vi "set current(without frequency).vi"(0 "源":i32, 5 "仪器设置":T2, 7 "电流":dbl, 9 "参考信号":T1, 11 "电阻":dbl) -> (10 "电压":dbl)   [LabVIEW 2019, in "old.lvlib"]
uses:
  lib/Keithley 622x/Configure/6221 Wave/Low Level/Typedefs/KE6221 -- Wave Type.ctl
  lib/Keithley 622x/Configure/6221 Wave/Low Level/Typedefs/KE6221 -- Wave Ranging Mode.ctl
  lib/Keithley 622x/Configure/6221 Wave/Low Level/Typedefs/KE6221 -- Wave Playback Time.ctl
  lib/Keithley 622x/Configure/Source/Typedefs/KE622x -- Current Level.ctl
  old.lvlib
  lib/Stanford Research 830/Stanford Research 830.lvlib
  lib/Keithley 622x/Keithley 622x.lvlib
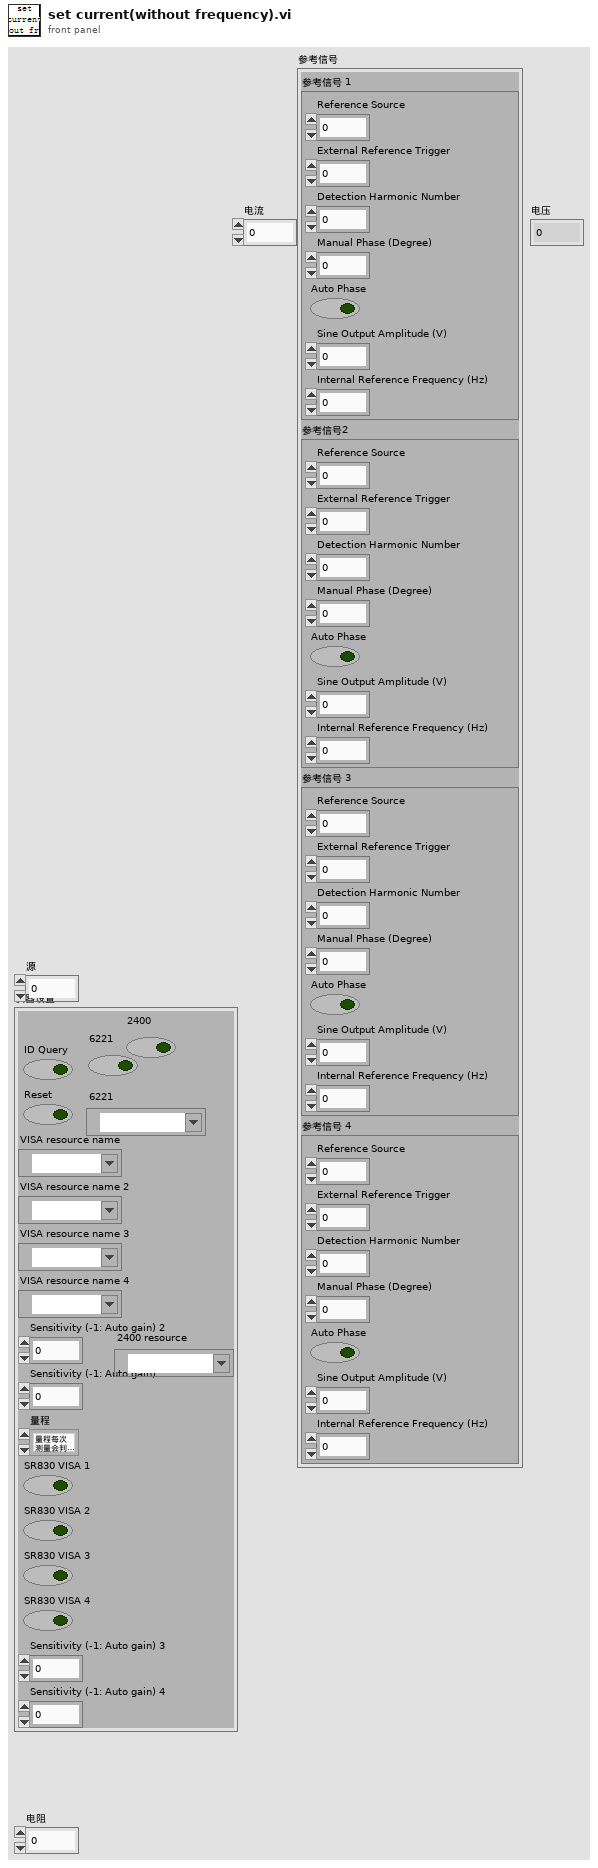
[diagram p1: front panel]
types:
  T1 = cluster{"参考信号 1":cluster{"Reference Source":u16, "External Reference Trigger  ":u16, "Detection Harmonic Number ":dbl, "Manual Phase (Degree)":dbl, "Auto Phase ":bool, "Sine Output Amplitude (V)":dbl, "Internal Reference Frequency (Hz)":dbl}, "参考信号2":cluster{"Reference Source":u16, "External Reference Trigger  ":u16, "Detection Harmonic Number ":dbl, "Manual Phase (Degree)":dbl, "Auto Phase ":bool, "Sine Output Amplitude (V)":dbl, "Internal Reference Frequency (Hz)":dbl}, "参考信号 3":cluster{"Reference Source":u16, "External Reference Trigger  ":u16, "Detection Harmonic Number ":dbl, "Manual Phase (Degree)":dbl, "Auto Phase ":bool, "Sine Output Amplitude (V)":dbl, "Internal Reference Frequency (Hz)":dbl}, "参考信号 4":cluster{"Reference Source":u16, "External Reference Trigger  ":u16, "Detection Harmonic Number ":dbl, "Manual Phase (Degree)":dbl, "Auto Phase ":bool, "Sine Output Amplitude (V)":dbl, "Internal Reference Frequency (Hz)":dbl}}
  T2 = cluster{"ID Query":bool, "Reset":bool, "VISA resource name":refnum<visa-resource-name>, "VISA resource name 2":refnum<visa-resource-name>, "VISA resource name 3":refnum<visa-resource-name>, "VISA resource name 4":refnum<visa-resource-name>, "Sensitivity (-1: Auto gain) 2":i16, "Sensitivity (-1: Auto gain)":i16, "量程":enum16{"量程每次测量会判定", "量程不变为设定值"}, "SR830 VISA 1":bool, "SR830 VISA 2":bool, "SR830 VISA 3":bool, "SR830 VISA 4":bool, "Sensitivity (-1: Auto gain) 3":i16, "Sensitivity (-1: Auto gain) 4":i16, "6221":bool, "6221":refnum<visa-resource-name>, "2400":bool, "2400 resource":refnum<visa-resource-name>}
  T3 = cluster{"Reference Source":u16, "External Reference Trigger  ":u16, "Detection Harmonic Number ":dbl, "Manual Phase (Degree)":dbl, "Auto Phase ":bool, "Sine Output Amplitude (V)":dbl, "Internal Reference Frequency (Hz)":dbl}
  T4 = typedef "Keithley 622x.lvlib/KE622x -- Current Level.ctl" = dbl
  T5 = typedef "Keithley 622x.lvlib/KE6221 -- Wave Playback Time.ctl" = dbl
  T6 = typedef "Keithley 622x.lvlib/KE6221 -- Wave Ranging Mode.ctl" = enum16{"Best", "Fixed"}
  T7 = typedef "Keithley 622x.lvlib/KE6221 -- Wave Type.ctl" = enum16{"Sinusoid", "Square", "Ramp", "Arbitrary 0", "Arbitrary 1", "Arbitrary 2", "Arbitrary 3", "Arbitrary 4"}
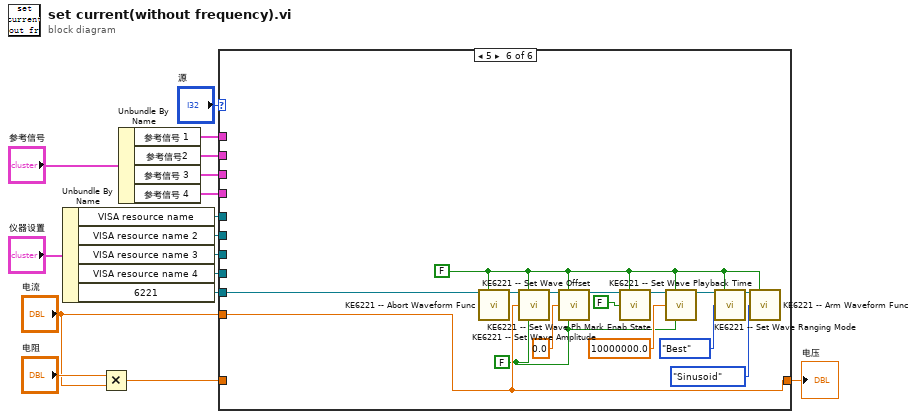
[diagram p0: block diagram]
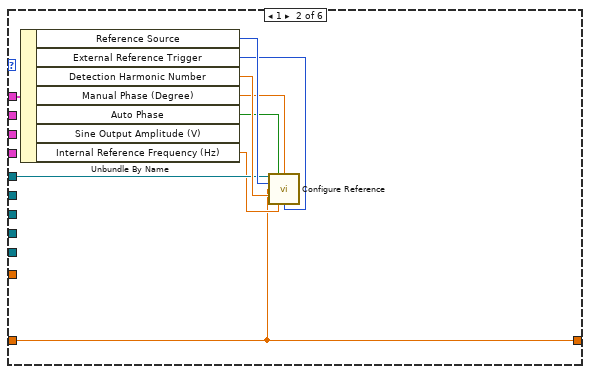
[diagram p3: hidden frame]
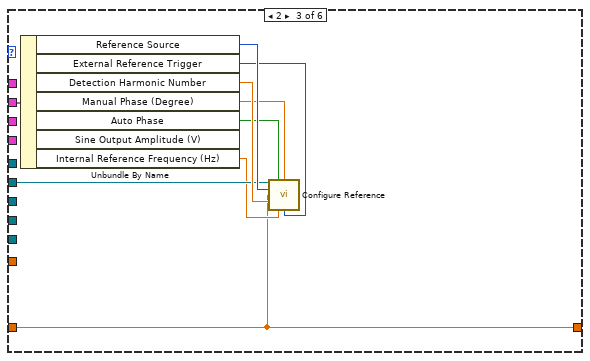
[diagram p4: hidden frame]
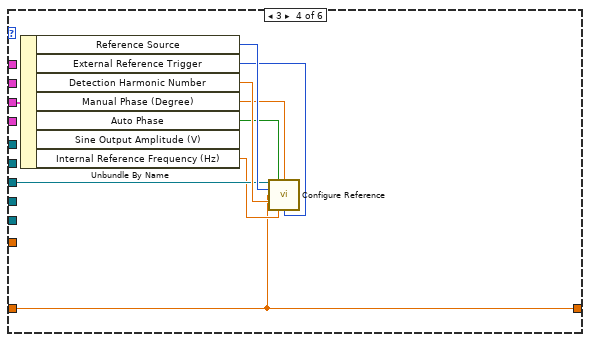
[diagram p5: hidden frame]
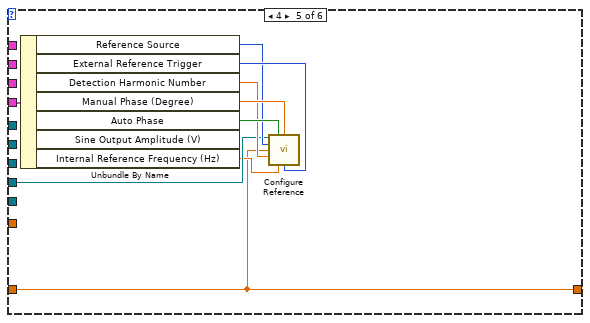
[diagram p6: hidden frame]
diagram:
  n1 = Unbundle By Name("仪器设置") -> ("VISA resource name"=w12:refnum<visa-resource-name>, "VISA resource name 2"=w15:refnum<visa-resource-name>, "VISA resource name 3"=w14:refnum<visa-resource-name>, "VISA resource name 4"=w13:refnum<visa-resource-name>, "6221"=w3:refnum<visa-resource-name>)
  n2 = Multiply(x="电阻", y="电流") -> (x*y=w11:dbl)
  n3 = Unbundle By Name("参考信号") -> ("参考信号 1"=w7:T3, "参考信号2"=w5:T3, "参考信号 3"=w4:T3, "参考信号 4"=w6:T3)
  n4 = case shown="5" "源" {
    tunnel: w11 -> [w17 w18 w27 w36 w45 _]
    tunnel: w12 -> [_ w21 _ _ _ _]
    tunnel: w13 -> [_ _ _ _ w48 _]
    tunnel: w14 -> [_ _ _ w39 _ _]
    tunnel: w15 -> [_ _ w30 _ _ _]
    tunnel: w7 -> [_ w20 _ _ _ _]
    tunnel: w5 -> [_ _ w29 _ _ _]
    tunnel: w4 -> [_ _ _ w38 _ _]
    tunnel: w6 -> [_ _ _ _ w47 _]
    tunnel: w3 -> [_ _ _ _ _ w66]
    tunnel: "电流" -> [_ _ _ _ _ w68]
    tunnel: [w17 w18 w27 w36 w45 w68] -> w1
    frame 0, Default {
    }
    frame 1 {
      n5 = Unbundle By Name(w20) -> ("Reference Source"=w26:u16, "External Reference Trigger"=w24:u16, "Detection Harmonic Number"=w25:dbl, "Manual Phase (Degree)"=w22:dbl, "Auto Phase"=w23:bool, "Internal Reference Frequency (Hz)"=w19:dbl)  [unwired: 1 out]
      n6 = call "Configure Reference.vi"("VISA resource name"=w21, "Auto Phase (T: Enabled)"=w23, "Manual Phase (0 Degree)"=w22, "Reference Source (1: Internal)"=w26, "Sine Output Amplitude (1 V)"=w18, "Detection Harmonic Number (1)"=w25, "Internal Reference Frequency (1000 Hz)"=w19, "External Reference Trigger (0: Sine Zero Crossing)"=w24) -> ()  [unwired: 6 in, 2 out]
    }
    frame 2 {
      n7 = Unbundle By Name(w29) -> ("Reference Source"=w35:u16, "External Reference Trigger"=w33:u16, "Detection Harmonic Number"=w34:dbl, "Manual Phase (Degree)"=w31:dbl, "Auto Phase"=w32:bool, "Internal Reference Frequency (Hz)"=w28:dbl)  [unwired: 1 out]
      n8 = call "Configure Reference.vi"("VISA resource name"=w30, "Auto Phase (T: Enabled)"=w32, "Manual Phase (0 Degree)"=w31, "Reference Source (1: Internal)"=w35, "Sine Output Amplitude (1 V)"=w27, "Detection Harmonic Number (1)"=w34, "Internal Reference Frequency (1000 Hz)"=w28, "External Reference Trigger (0: Sine Zero Crossing)"=w33) -> ()  [unwired: 6 in, 2 out]
    }
    frame 3 {
      n9 = Unbundle By Name(w38) -> ("Reference Source"=w44:u16, "External Reference Trigger"=w42:u16, "Detection Harmonic Number"=w43:dbl, "Manual Phase (Degree)"=w40:dbl, "Auto Phase"=w41:bool, "Internal Reference Frequency (Hz)"=w37:dbl)  [unwired: 1 out]
      n10 = call "Configure Reference.vi"("VISA resource name"=w39, "Auto Phase (T: Enabled)"=w41, "Manual Phase (0 Degree)"=w40, "Reference Source (1: Internal)"=w44, "Sine Output Amplitude (1 V)"=w36, "Detection Harmonic Number (1)"=w43, "Internal Reference Frequency (1000 Hz)"=w37, "External Reference Trigger (0: Sine Zero Crossing)"=w42) -> ()  [unwired: 6 in, 2 out]
    }
    frame 4 {
      n11 = Unbundle By Name(w47) -> ("Reference Source"=w49:u16, "External Reference Trigger"=w51:u16, "Detection Harmonic Number"=w50:dbl, "Manual Phase (Degree)"=w53:dbl, "Auto Phase"=w52:bool, "Internal Reference Frequency (Hz)"=w46:dbl)  [unwired: 1 out]
      n12 = call "Configure Reference.vi"("VISA resource name"=w48, "Auto Phase (T: Enabled)"=w52, "Manual Phase (0 Degree)"=w53, "Reference Source (1: Internal)"=w49, "Sine Output Amplitude (1 V)"=w45, "Detection Harmonic Number (1)"=w50, "Internal Reference Frequency (1000 Hz)"=w46, "External Reference Trigger (0: Sine Zero Crossing)"=w51) -> ()  [unwired: 6 in, 2 out]
    }
    frame 5 {
      w60 = FALSE ("Check For SCPI Errors? (T)")
      w54 = FALSE ("Read Back Set Value? (T)")
      n13 = call "KE6221 -- Abort Waveform Func.vi"("Resource In"=w66, "Check For SCPI Errors? (T)"=w60) -> ("Resource Out (dupl)"=w67:refnum<visa-resource-name>)  [unwired: 12 in, 1 out]
      n14 = call "KE6221 -- Set Wave Amplitude.vi"("Resource In"=w67, "Check For SCPI Errors? (T)"=w60, "Wave Amplitude In"=w68, "Read Back Set Value? (T)"=w54) -> ("Resource Out (dupl)"=w65:refnum<visa-resource-name>)  [unwired: 9 in, 2 out]
      n15 = call "KE6221 -- Set Wave Offset.vi"("Resource In"=w65, "Check For SCPI Errors? (T)"=w60, "Wave Offset In (A)"=T4 0.0, "Read Back Set Value? (T)"=w54) -> ("Resource Out (dupl)"=w64:refnum<visa-resource-name>)  [unwired: 9 in, 2 out]
      n16 = call "KE6221 -- Set Wave Ph Mark Enab State.vi"("Resource In"=w64, "Check For SCPI Errors? (T)"=w60, "Phase Marker Enabled?"=FALSE) -> ("Resource Out (dupl)"=w63:refnum<visa-resource-name>)  [unwired: 11 in, 1 out]
      n17 = call "KE6221 -- Set Wave Playback Time.vi"("Resource In"=w63, "Check For SCPI Errors? (T)"=w60, "Playback Time (s) In"=T5 10000000.0, "Read Back Set Value? (T)"=w54) -> ("Resource Out (dupl)"=w62:refnum<visa-resource-name>)  [unwired: 9 in, 2 out]
      n18 = call "KE6221 -- Set Wave Ranging Mode.vi"("Resource In"=w62, "Check For SCPI Errors? (T)"=w60, "Ranging Mode"=KE6221_--_Wave_Ranging_Mode."Best") -> ("Resource Out (dupl)"=w61:refnum<visa-resource-name>)  [unwired: 11 in, 1 out]
      n19 = call "KE6221 -- Arm Waveform Func.vi"("Resource In"=w61, "Check For SCPI Errors? (T)"=w60, "Wave Type"=KE6221_--_Wave_Type."Sinusoid") -> ()  [unwired: 11 in, 2 out]
    }
  }
  "电压" <- w1
